vi "Initialize 6R Type 2 Serial Arm.vi"(8 "error in (no error)":errorcluster, 10 "dynamic parameters":T1[](array[typedef]), 11 "kinematic parameters":T3[](array[typedef])) -> (0 "error out":errorcluster, 3 "6R type 2 serial arm out":refnum<class "NI_Robotics_6R Type 2 Serial Arm Class.lvclass">)   [LabVIEW 2017, in "NI_Robotics_6R Type 2 Serial Arm Class.lvclass"]
doc: "Sets the properties of a serial robot arm and generates a representation of the arm. If you have access to a 6R, 5R, or SCARA arm, generate that type of arm. If you do not have access to an arm of those types, generate a generic arm. You must manually select the polymorphic instance to use."
uses:
  <vilib>/robotics/Kinematics/Analytical/6R/Type 2/NI_Robotics_6R Type 2 Serial Arm Class.lvclass
  c:/Program Files (x86)/National Instruments/LabVIEW 2017/vi.lib/robotics/Kinematics/Robot/NI_Robotics_Serial Robot Arm.lvclass
  <vilib>/robotics/Kinematics/DH Kinematic Parameters.ctl
  <vilib>/robotics/Kinematics/Link/Joint Type.ctl
  <vilib>/robotics/Kinematics/DH Dynamic Parameters.ctl
  <vilib>/Analysis/Matrix/Datatypes/RealMatrix.ctl
  <vilib>/robotics/Kinematics/Link/NI_Robotics_Link.lvclass
  <vilib>/robotics/Kinematics/Robot/NI_Robotics_Serial Robot Arm.lvclass
  <vilib>/robotics/Utilities/NI_Robotics Utilities.lvlib
  <vilib>/Analysis/Matrix/NI_Matrix.lvlib
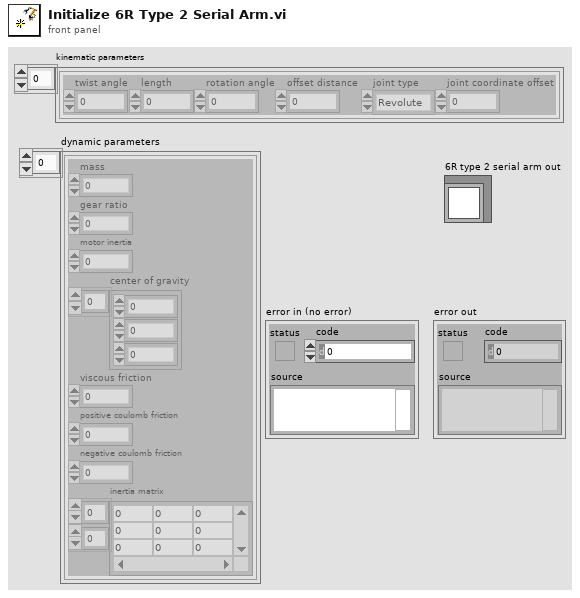
[diagram p1: front panel]
types:
  T1 = typedef "DH Dynamic Parameters.ctl" = cluster{"mass":dbl, "gear ratio":dbl, "motor inertia":dbl, "center of gravity":dbl[], "viscous friction":dbl, "positive coulomb friction":dbl, "negative coulomb friction":dbl, "inertia matrix":T2}
  T2 = typedef "NI_Matrix.lvlib/RealMatrix.ctl" = dbl[][]
  T3 = typedef "DH Kinematic Parameters.ctl" = cluster{"twist angle":dbl, "length":dbl, "rotation angle":dbl, "offset distance":dbl, "joint type":T4, "joint coordinate offset":dbl}
  T4 = typedef "NI_Robotics_Link.lvclass/Joint Type.ctl" = enum16{"Revolute", "Prismatic"}
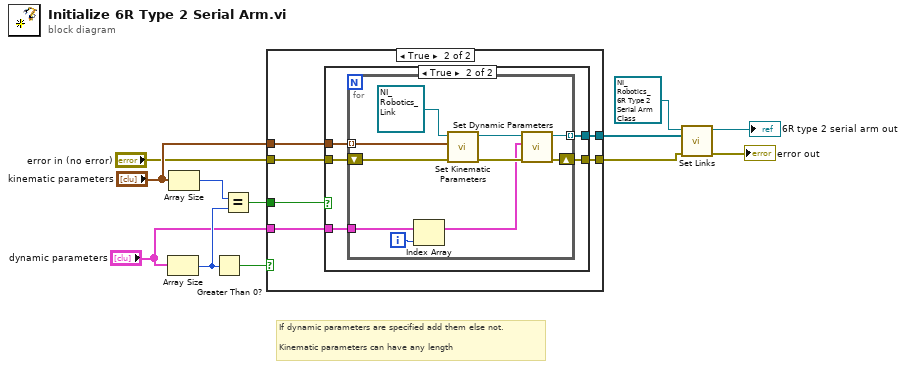
[diagram p0: block diagram]
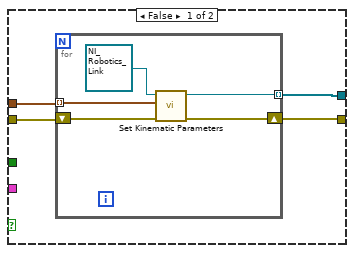
[diagram p2: hidden frame]
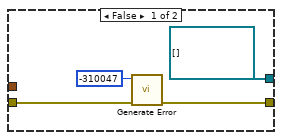
[diagram p3: hidden frame]
diagram:
  # "If dynamic parameters are specified add them else not.\n\nKinematic parameters can have any length"
  n1 = Array Size(array="dynamic parameters") -> (size(s)=w7:i32)
  n2 = Array Size(array="kinematic parameters") -> (size(s)=w8:i32)
  n3 = Greater Than 0?(x=w7) -> (x > 0?=w9:bool)
  n4 = Equal?(x=w8, y=w7) -> (x = y?=w6:bool)
  n5 = case shown="True" w9 {
    tunnel: "kinematic parameters" -> [w16 w27]
    tunnel: "error in (no error)" -> [w15 w26]
    tunnel: [w13 w25] -> w4
    tunnel: [w14 w24] -> w5
    tunnel: "dynamic parameters" -> [_ w23]
    tunnel: w6 -> [_ w22]
    frame False {
      n6 = for {
        tunnel: w16 -> [w20] mode=indexing
        shift-right: [w17] -> w13
        shift-left: w15 -> [w19]
        tunnel: [w18] -> w14 mode=indexing
        n7 = call <vilib>:"Set Kinematic Parameters.vi"("error in (no error)"=w19, "kinematic parameters"=w20, "link in"=refnum<class "NI_Robotics_Link.lvclass"> refnum ("Link")) -> ("error out"=w17:errorcluster, "link out"=w18:refnum<class "NI_Robotics_Link.lvclass">)  [unwired: 7 in]
      }
    }
    frame True {
      n8 = case shown="True" w22 {
        tunnel: w27 -> [_ w36]
        tunnel: w26 -> [w29 w35]
        tunnel: [w30 w34] -> w25
        tunnel: [refnum<class "NI_Robotics_Link.lvclass">[] [] w33] -> w24
        tunnel: w23 -> [_ w32]
        frame False {
          n9 = call <vilib>:"Generate Error.vi"("error in (no error)"=w29, "code"=-310047) -> ("error out"=w30:errorcluster)  [unwired: 9 in]
        }
        frame True {
          n10 = for {
            tunnel: w36 -> [w45] mode=indexing
            tunnel: w32 -> [w42]
            tunnel: [w40] -> w33 mode=indexing
            shift-right: [w41] -> w34
            shift-left: w35 -> [w39]
            i -> [w37]
            n11 = Index Array(array=w42, index=w37) -> (element=w38:T1)
            n12 = call <vilib>:"Set Kinematic Parameters.vi"("error in (no error)"=w39, "kinematic parameters"=w45, "link in"=refnum<class "NI_Robotics_Link.lvclass"> refnum ("Link")) -> ("error out"=w43:errorcluster, "link out"=w44:refnum<class "NI_Robotics_Link.lvclass">)  [unwired: 7 in]
            n13 = call <vilib>:"Set Dynamic Parameters.vi"("error in (no error)"=w43, "dynamic parameters"=w38, "link in"=w44) -> ("error out"=w41:errorcluster, "link out"=w40:refnum<class "NI_Robotics_Link.lvclass">)  [unwired: 7 in]
          }
        }
      }
    }
  }
  n14 = call <vilib>:"Set Links.vi"("error in (no error)"=w4, "links"=w5, "serial arm in"=refnum<class "NI_Robotics_6R Type 2 Serial Arm Class.lvclass"> refnum ("6R Type 2 Serial Arm Class out")) -> ("error out"=→"error out":errorcluster, "serial arm out"=→"6R type 2 serial arm out":refnum<class "NI_Robotics_6R Type 2 Serial Arm Class.lvclass">)  [unwired: 7 out]
